vi "Proyecto Final completo.vi"() -> ()   [LabVIEW 2020]
uses:
  <vilib>/Instr/_visa.llb/VISA Configure Serial Port (Instr).vi
panel:
  out "error out":errorcluster
  in  "Tab Control":enum16{""}(ring)
  out "Encoder":dbl
  out "Movimiento lineal":dbl
  out "Proximidad":dbl
  out "Intensidad de luz":dbl
  out "Peso":dbl
  out "Velocidad del viento":dbl
  out "Humedad Relativa":dbl
  out "Corriente DC":dbl
  out "Voltaje DC":dbl
  out "Corriente AC":dbl
  out "Voltaje AC":dbl
  out "Electronico":dbl
  out "read buffer 2":string
  out "Termistor":dbl
  out "length":i32
  in  "Tamaño de  comparacion":i32
  out "Termocopla":dbl(graph)
  out "RTD":dbl
  out "Serial Settings:Number of Bytes at Serial Port":u32
  in  "millisecond multiple":u32
  in  "STOP":bool
  out "read buffer":string
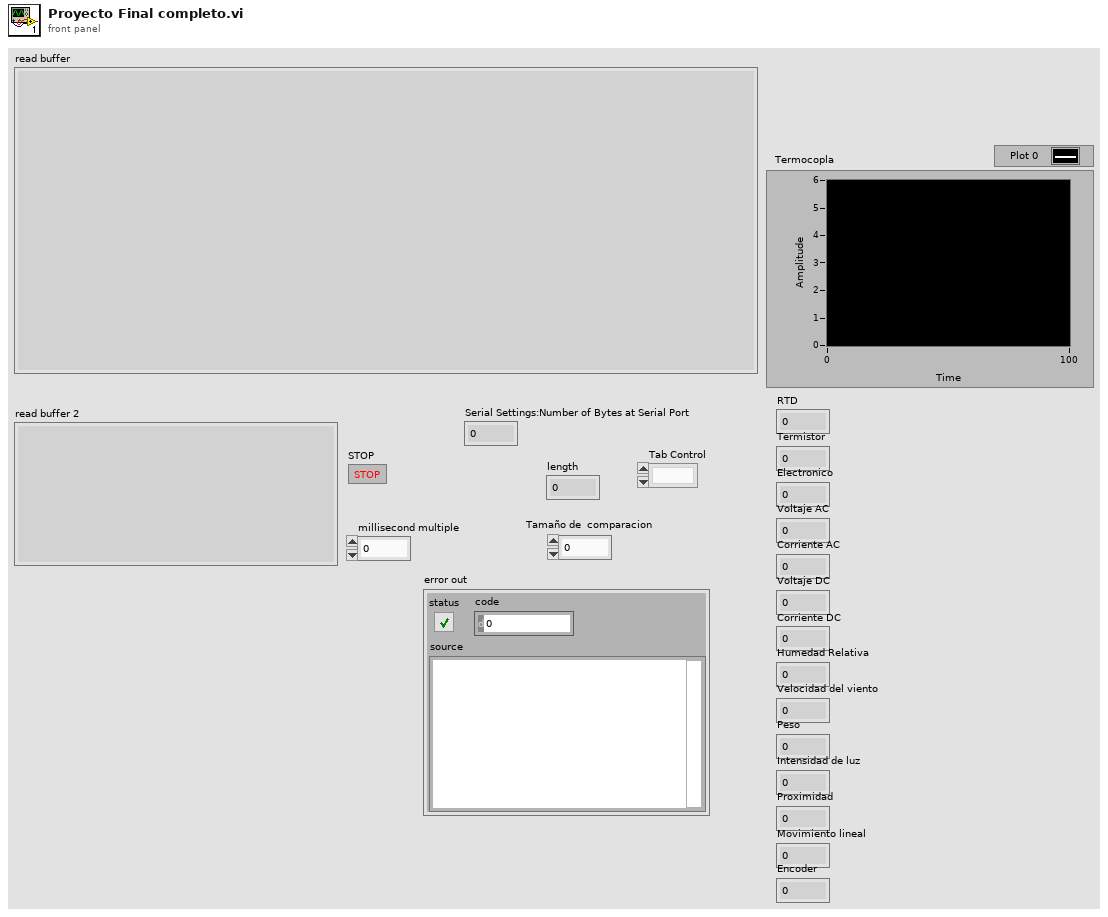
[diagram p1: front panel]
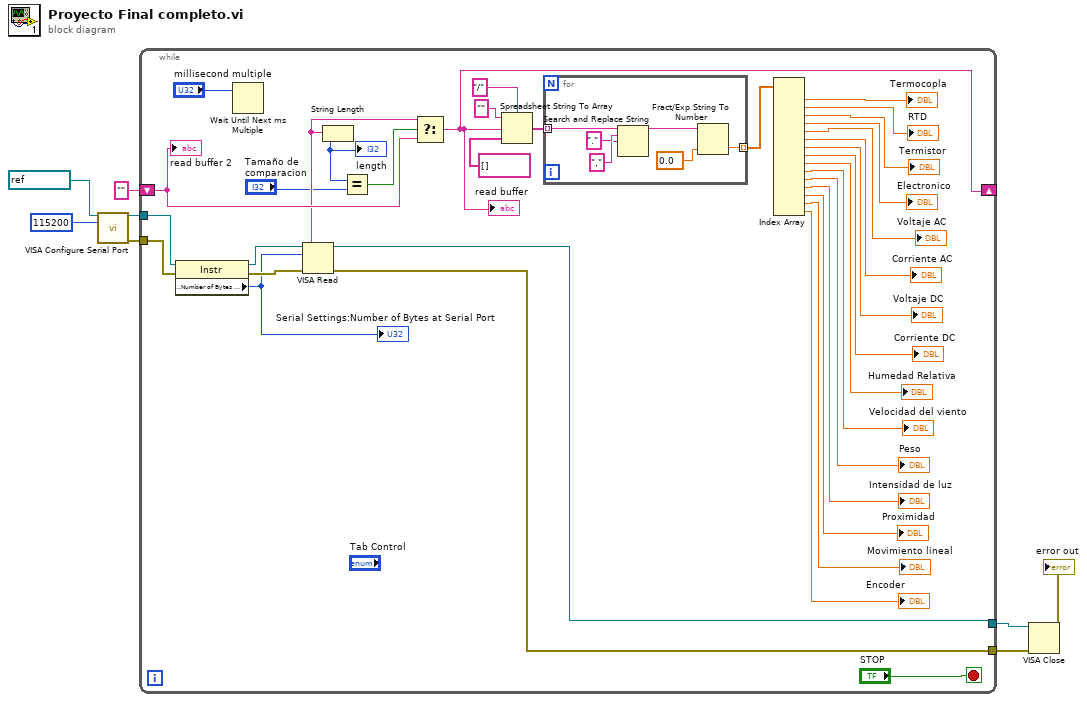
[diagram p0: block diagram]
diagram:
  n1 = call-poly "VISA Configure Serial Port"("VISA resource name"=refnum<visa-resource-name> "COM3", "baud rate (9600)"=u32 115200) -> ("VISA resource name out"=w6:refnum<visa-resource-name>, "error out"=w5:errorcluster)  [unwired: 12 in]
  n2 = while {
    tunnel: w6 -> [w43]
    tunnel: w5 -> [w42]
    tunnel: [w38] -> w4
    tunnel: [w37] -> w3
    shift-right: [w12] -> _
    shift-left: "" ("read buffer") -> [w28]
    stop <- "STOP" stop-if-true
    n3 = property class="Instr"(reference=w43, error in=w42) -> (reference out=w41:refnum<visa-resource-name>, error out=w40:errorcluster, "Serial Settings:Number of Bytes at Serial Port"=w39:u32)
    "Serial Settings:Number of Bytes at Serial Port" <- w39
    n4 = Wait Until Next ms Multiple(millisecond multiple="millisecond multiple") -> ()  [unwired: 1 out]
    n5 = VISA Read(VISA resource name=w41, byte count=w39, error in (no error)=w40) -> (VISA resource name out=w38:refnum<visa-resource-name>, read buffer=w13:string, error out=w37:errorcluster)  [unwired: 1 out]
    n6 = String Length(string=w13) -> (length=w11:i32)
    "length" <- w11
    n7 = Equal?(x=w11, y="Tamaño de  comparacion") -> (x = y?=w9:bool)
    n8 = Select(t=w13, s=w9, f=w28) -> (s? t:f=w12:string)
    "read buffer" <- w12
    n9 = Spreadsheet String To Array(delimiter (Tab)="/", format string="", spreadsheet string=w12, array type (2D Dbl)=string[] []) -> (array=w31:string[])
    n10 = for {
      tunnel: w31 -> [w49] mode=indexing
      tunnel: [w44] -> w30 mode=indexing
      n11 = Search and Replace String(input string=w49, search string=".", replace string="," ("replace string (\"\")")) -> (result string=w46:string)  [unwired: 5 in, 3 out]
      n12 = Fract/Exp String To Number(string=w46, default (0 dbl)=0.0 ("default (0 DBL)")) -> (number=w44:dbl)  [unwired: 2 in, 1 out]
    }
    n13 = Index Array(array=w30) -> (element #1=→"Termocopla":dbl, element #2=→"RTD":dbl, element #3=→"Termistor":dbl, element #4=→"Electronico":dbl, element #5=→"Voltaje AC":dbl, element #6=→"Corriente AC":dbl, element #7=→"Voltaje DC":dbl, element #8=→"Corriente DC":dbl, element #9=→"Humedad Relativa":dbl, element #10=→"Velocidad del viento":dbl, element #11=→"Peso":dbl, element #12=→"Intensidad de luz":dbl, element #13=→"Proximidad":dbl, element #14=→"Movimiento lineal":dbl, element #15=→"Encoder":dbl)  [unwired: 15 in]
    "read buffer 2" <- w28
  }
  n14 = VISA Close(VISA resource name=w4, error in (no error)=w3) -> (error out=→"error out":errorcluster)
